vi "Interpolate Analog Inputs.vi"(8 "error in (no error)":errorcluster, 11 "Hardware Interface in":refnum<class "Hardware Interface.lvclass">) -> (0 "error out":errorcluster, 2 "Interpolated Values":dbl[](array[numeric]), 3 "Hardware Interface out":refnum<class "Hardware Interface.lvclass">)   [LabVIEW 2013, in "Hardware Interface.lvclass"]
uses:
  Hardware Interface.lvclass
  Hardware Interface.lvclass/Hardware Interface.ctl
  <vilib>/Analysis/polynomials.llb/Scalar Polynomial Evaluation (DBL).vi
  <vilib>/Analysis/NI_AALPro.lvlib
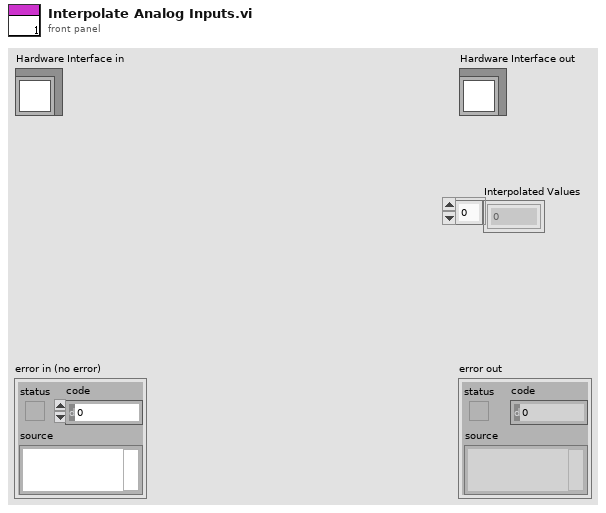
[diagram p1: front panel]
types:
  T1 = typedef "NI_Matrix.lvlib/RealMatrix.ctl" = dbl[][]
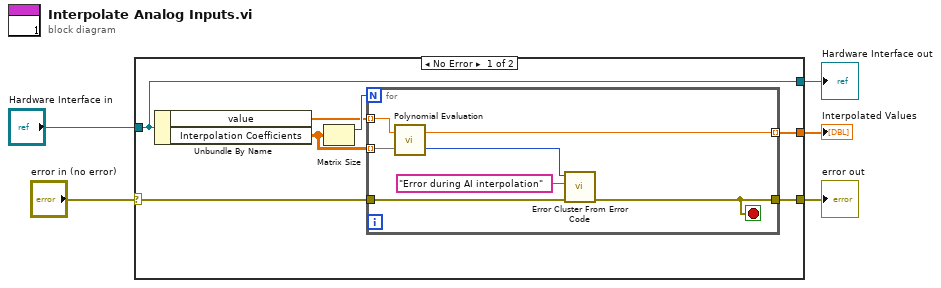
[diagram p0: block diagram]
diagram:
  n1 = case shown="No Error" "error in (no error)" {
    selector: "error in (no error)" -> [w7 w21]
    tunnel: [w6 w21] -> w4
    tunnel: [w12 w20] -> w2
    tunnel: "Hardware Interface in" -> [w12 w20]
    tunnel: [w8 _] -> w1
    frame No Error {
      n2 = Unbundle By Name(w12) -> ("value"=w9:dbl[], "Interpolation Coefficients"=w10:T1)
      n3 = Matrix Size(0:w10) -> (1:w11:i32)  [unwired: 1 out]
      n4 = for {
        N: w11 -> [_]
        tunnel: w10 -> [w19] mode=indexing
        tunnel: w9 -> [w18] mode=indexing
        tunnel: [w17] -> w8 mode=indexing
        tunnel: w7 -> [w15]
        tunnel: [w14] -> w6
        stop <- w14 stop-if-true
        n5 = call-poly <vilib>:"Polynomial Evaluation.vi"("P(x)"=w19, "a"=w18) -> ("error"=w16:i32, "P(a)"=w17:dbl)
        n6 = call <vilib>:"Error Cluster From Error Code.vi"("error in (no error)"=w15, "error message (\"\")"="Error during AI interpolation" ("error message (\"\")"), "error code (0)"=w16) -> ("error out"=w14:errorcluster)  [unwired: 6 in]
      }
    }
    frame Error {
    }
  }
  "error out" <- w4
  "Hardware Interface out" <- w2
  "Interpolated Values" <- w1
